vi "oa_Build DC Output Data (1 Channel).vi"(0 "DC value out":dbl[](array[numeric]), 1 "reset? (True)":bool=TRUE, 2 "X axis selection":u16(ring)=2 items=["Time", "Revolution", "RPM"], 5 "start points":dbl[](array[numeric]) format="%.2f", 7 "channel info":T1={"sensor sensitivity"=1000.0, "engineering units"=1, "dB reference"=1.0, "custom label"="EU", "weighting filter"=0, "pregain"=0.0} {"pregain" format="%.2f"; "weighting filter" items=["Linear", "A-weighting", "B-weighting", "C-weighting", "ITU-R 468-4", "Dolby", "CCITT", "C-message", "Wb", "Wc", "Wd", "We", "Wf", "Wh", "Wj", "Wk", "Wm", "AES17 20 kHz lowpass", "AES17 40 kHz lowpass", "AES17 20 kHz highpass", "AES17 40 kHz highpass"]; "dB reference" format="%^.1e"; "engineering units" items=["custom..."=0, "V"=1, "A"=21, "C"=30, "pC"=31, "s"=32, "-"=29, "Pa"=2, "N"=20, "g"=3, "m/s^2"=4, "m/s"=5, "m"=6, "mm/s"=12, "mm"=13, "micron/s"=14, "micron"=15, "in/s^2"=7, "in/s"=8, "in"=9, "mil/s"=10, "mil"=11, "rad/s^2"=16, "rad/s"=17, "rad"=18, "deg/s^2"=26, "deg/s"=27, "deg"=28, "RPM"=22, "cycle/s^2"=23, "Hz"=24, "cycle"=25, "strain"=19]; "sensor sensitivity" format="%#_5f"}, 9 "samples/rev":dbl, 11 "error in (no error)":errorcluster, 12 "DC gap unit":u16(ring) items=["V", "EU"]) -> (4 "DC Gap":cluster{"X":dbl[], "Y":dbl[]} {"Y" format="%.2f"; "X" format="%.2f"}, 8 "unit labels":cluster{"X unit":string, "gap unit":string}, 10 "DC gap positions [s]":dbl[](array[numeric]) format="%.2f", 15 "error out":errorcluster)   [LabVIEW 2017, in "SoundVib_RefDataProcess.lvlib"]
uses:
  <vilib>/addons/Sound and Vibration/Order Analysis/Referece Data Processing/SoundVib_RefDataProcess.lvlib
  <vilib>/addons/_NISVFA/_Shared subVIs/Controls/svc_Channel Info.ctl
  <vilib>/addons/_NISVFA/_Shared subVIs/Controls/svc_Engineering Units Text Ring.ctl
  <vilib>/addons/_NISVFA/_Shared subVIs/Controls/svc_Weighting Filter Text Ring.ctl
  <vilib>/Analysis/1siggen.llb/Ramp Pattern by Samples.vi
  <vilib>/addons/Sound and Vibration/Order Analysis/Resample Order Tracking/SoundVib_Resampling.lvlib
  <vilib>/Analysis/NI_AALBase.lvlib
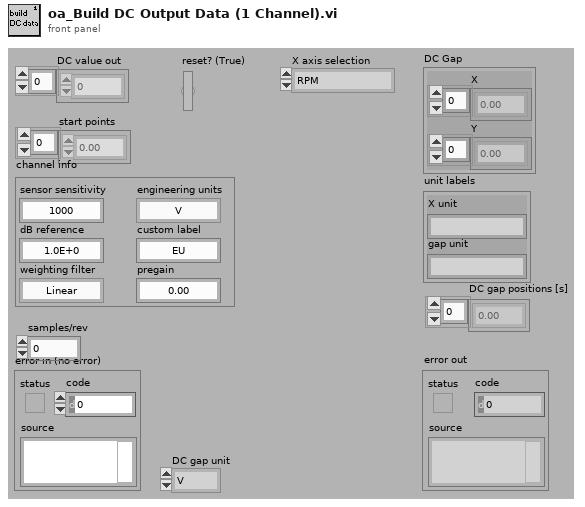
[diagram p1: front panel]
types:
  T1 = typedef "svc_Channel Info.ctl" = cluster{"sensor sensitivity":dbl, "engineering units":T2, "dB reference":dbl, "custom label":string, "weighting filter":T3, "pregain":dbl}
  T2 = typedef "svc_Engineering Units Text Ring.ctl" = u16
  T3 = typedef "svc_Weighting Filter Text Ring.ctl" = u16
  T4 = typedef "SoundVib_TachProcess.lvlib/speed profile.ctl" = cluster{"time [s]":dbl[], "speed [RPM]":dbl[]}
  T5 = cluster{"speed [RPM]":dbl[], "DC value out":dbl[]}
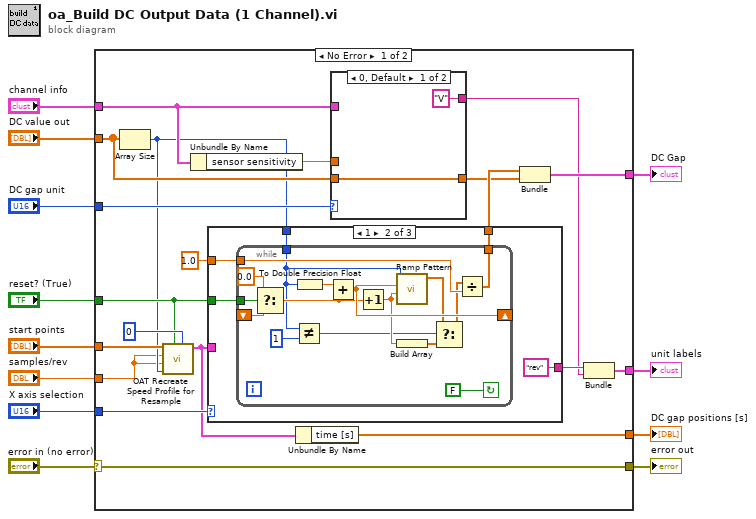
[diagram p0: block diagram]
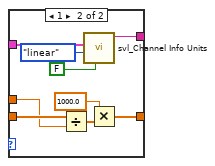
[diagram p2: hidden frame]
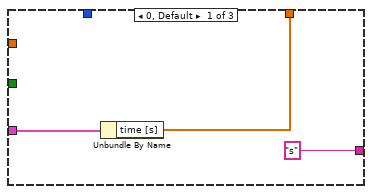
[diagram p3: hidden frame]
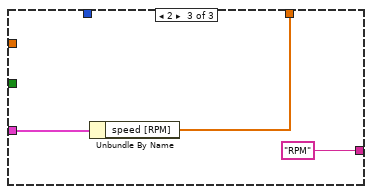
[diagram p4: hidden frame]
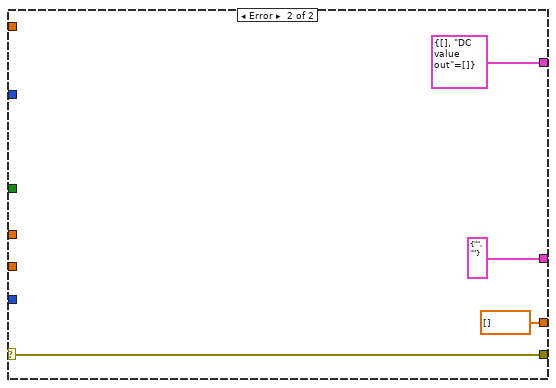
[diagram p5: hidden frame]
diagram:
  n1 = case shown="No Error" "error in (no error)" {
    selector: "error in (no error)" -> [w25 w74]
    tunnel: "X axis selection" -> [w29 _]
    tunnel: "reset? (True)" -> [w28 _]
    tunnel: [w27 cluster{dbl[], "DC value out":dbl[]} {[], "DC value out"=[]}] -> w10
    tunnel: "DC value out" -> [w15 _]
    tunnel: "start points" -> [w26 _]
    tunnel: [w25 w74] -> w6
    tunnel: [w23 cluster{string, "unit label":string} {"", "unit label"=""}] -> w5
    tunnel: "channel info" -> [w19 _]
    tunnel: "DC gap unit" -> [w22 _]
    tunnel: [w16 dbl[] [] ("time [s]")] -> w2
    tunnel: "samples/rev" -> [w13 _]
    frame No Error {
      n2 = Array Size(array=w15) -> (size(s)=w14:i32)
      n3 = call <vilib>:"OAT Recreate Speed Profile for Resample.vi"("lags"=0, "init/continue (init:T)"=w28, "output length"=w14, "decimation factor"=w13, "sample / rev"=w13, "time stamps in"=w26) -> ("speed profile"=w17:T4)  [unwired: 5 in]
      n4 = Unbundle By Name(w19) -> ("sensor sensitivity"=w20:dbl)
      n5 = case shown="1" w29 {
        tunnel: w17 -> [w46 _ w70]
        tunnel: [w45 w51 w69] -> w31
        tunnel: w14 -> [_ w48 _]
        tunnel: 1.0 ("samples/rev") -> [_ w50 _]
        tunnel: w28 -> [_ w49 _]
        tunnel: ["s" "rev" "RPM"] -> w24
        frame 0, Default {
          n6 = Unbundle By Name(w46) -> ("time [s]"=w45:dbl[])
        }
        frame 1 {
          n7 = while {
            tunnel: [w67] -> w51
            tunnel: w50 -> [w66]
            tunnel: w49 -> [w64]
            shift-right: [w61] -> _
            shift-left: _ -> [w62]
            tunnel: w48 -> [w58]
            stop <- FALSE continue-if-true
            n8 = Select(t=0.0 ("f"), s=w64, f=w62) -> (s? t:f=w60:dbl)
            n9 = Not Equal?(x=w58, y=1) -> (x != y?=w56:bool)
            n10 = To Double Precision Float(number=w58) -> (double precision float=w52:dbl)
            n11 = Add(x=w52, y=w60) -> (x+y=w61:dbl)
            n12 = Increment(x=w60) -> (x+1=w57:dbl)
            n13 = call-poly <vilib>:"Ramp Pattern.vi"("start"=w57, "end"=w61, "samples"=w58) -> ("Ramp Pattern"=w55:dbl[])  [unwired: 7 in, 1 out]
            n14 = Build Array(w57) -> (w54:dbl[])
            n15 = Select(t=w55, s=w56, f=w54) -> (s? t:f=w53:dbl[])
            n16 = Divide(x=w53, y=w66) -> (x/y=w67:dbl[])
          }
        }
        frame 2 {
          n17 = Unbundle By Name(w70) -> ("speed [RPM]"=w69:dbl[])
        }
      }
      n18 = Unbundle By Name(w17) -> ("time [s]"=w16:dbl[])
      n19 = case shown="0, Default" w22 {
        tunnel: w15 -> [w34 w43]
        tunnel: [w34 w39] -> w21
        tunnel: w20 -> [_ w42]
        tunnel: w19 -> [_ w36]
        tunnel: ["V" ("unit label") w35] -> w18
        frame 0, Default {
        }
        frame 1 {
          n20 = Divide(x=w43, y=w42) -> (x/y=w41:dbl[])
          n21 = call <vilib>:"svl_Channel Info Units.vi"("include weighting if dB On FALSE"=FALSE, "linear/dB"=enum16{"linear", "dB"}."linear", "channel info"=w36) -> ("unit label"=w35:string)  [unwired: 7 in, 1 out]
          n22 = Multiply(x=1000.0, y=w41) -> (x*y=w39:dbl[])
        }
      }
      n23 = Bundle("speed [RPM]"=w31, "DC value out"=w21) -> (w27:T5)  [unwired: 1 in]
      n24 = Bundle(w24, "unit label"=w18) -> (w23:cluster{string, "unit label":string})  [unwired: 1 in]
    }
    frame Error {
    }
  }
  "error out" <- w6
  "DC Gap" <- w10
  "unit labels" <- w5
  "DC gap positions [s]" <- w2
